vi "LWXPS_PositionerMotionDoneGet.vi"(0 "XPS Reference IN":refnum<k24>, 7 "Positioner Name":string, 11 "LabVIEW error IN":errorcluster) -> (2 "XPS Reference OUT":refnum<k24>, 3 "Returned error code":i32, 4 "Position window":dbl, 6 "Velocity window":dbl, 8 "Checking time":dbl, 10 "Mean period":dbl, 13 "LabVIEW error OUT":errorcluster, 14 "XPS Error String":string, 15 "Motion done time out":dbl)   [LabVIEW 2014]
uses:
  D:/XPSQ8_LabView_Library/Development/Source/Dll/Newport.XPS.CommandInterface.dll
  Dll/Newport.XPS.CommandInterface.dll
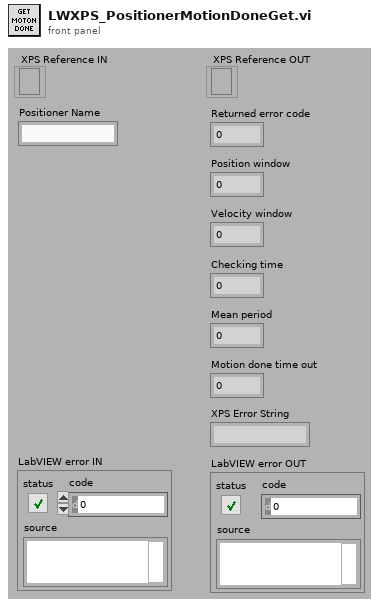
[diagram p1: front panel]
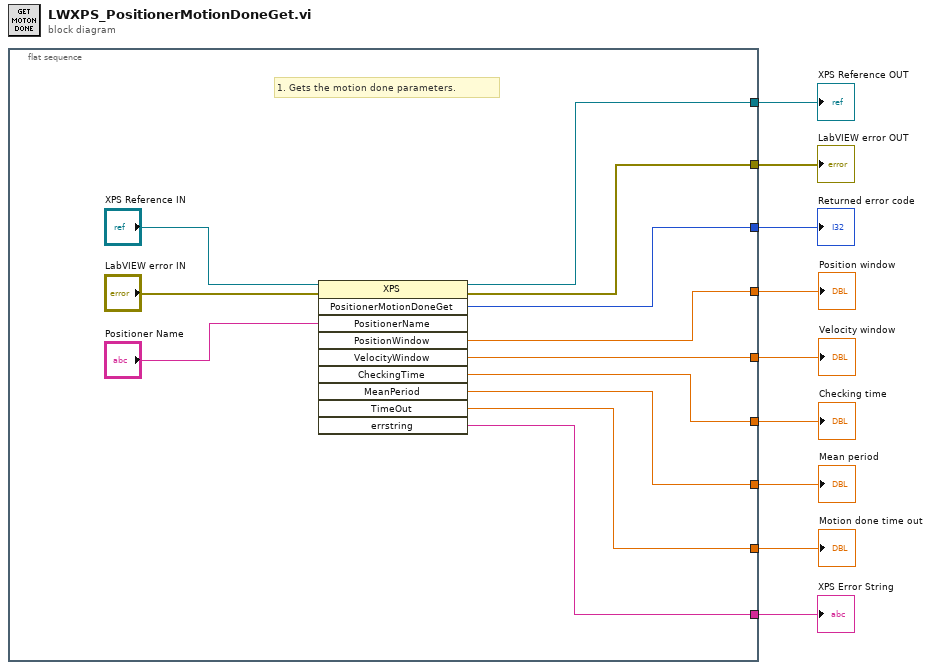
[diagram p0: block diagram]
diagram:
  n1 = flat-sequence {
    tunnel: [w15] -> w1
    tunnel: [w20] -> w9
    tunnel: [w19] -> w8
    tunnel: [w18] -> w7
    tunnel: [w14] -> w5
    tunnel: [w13] -> w4
    tunnel: [w12] -> w3
    tunnel: [w11] -> w2
    tunnel: [w10] -> w6
    frame #0 {
      # "1. Gets the motion done parameters."
      n2 = invoke class="XPS" method="PositionerMotionDoneGet"(reference="XPS Reference IN", error in="LabVIEW error IN", "PositionerName"="Positioner Name") -> (reference out=w20:refnum<k24>, error out=w19:errorcluster, "PositionerMotionDoneGet"=w18:i32, "PositionWindow"=w15:dbl, "VelocityWindow"=w14:dbl, "CheckingTime"=w13:dbl, "MeanPeriod"=w12:dbl, "TimeOut"=w11:dbl, "errstring"=w10:string)  [unwired: 7 in, 1 out]
    }
  }
  "XPS Error String" <- w6
  "XPS Reference OUT" <- w9
  "LabVIEW error OUT" <- w8
  "Returned error code" <- w7
  "Velocity window" <- w5
  "Checking time" <- w4
  "Mean period" <- w3
  "Motion done time out" <- w2
  "Position window" <- w1
